vi "Redirect Versions in Deployment Project File.vi"() -> ()   [LabVIEW 2013, in "Assembly Redirection VIs.lvlib"]
uses:
  Assembly Redirection VIs.lvlib
panel:
  in  "New TestStand Registry Version":string="5.1"
  in  "New VeriStand Version":string="2013"
  in  "destination file path":path=path "C:/Users/achurch/Documents/Source/XML Assembly Redirection Project/Examples XML Files/VeristandStepsInstaller_mod.vdproj"
  out "error out":errorcluster
  in  "New TestStand Version":string="2013"
  in  "configuration file path":path=path "C:/Users/achurch/Documents/Source/XML Assembly Redirection Project/Examples XML Files/VeristandStepsInstaller.vdproj"
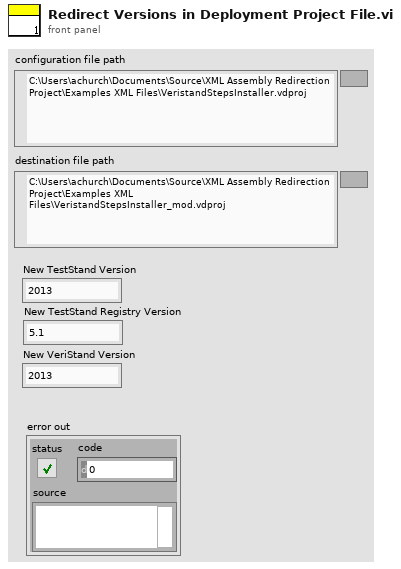
[diagram p1: front panel]
types:
  T1 = enum16{"open", "replace", "create", "open or create", "replace or create", "replace or create with confirmation"}
  T2 = enum32{"invalid app kind", "Development System", "Run Time System", "Student Edition", "Embedded LabVIEW", "Evaluation", "Custom"}
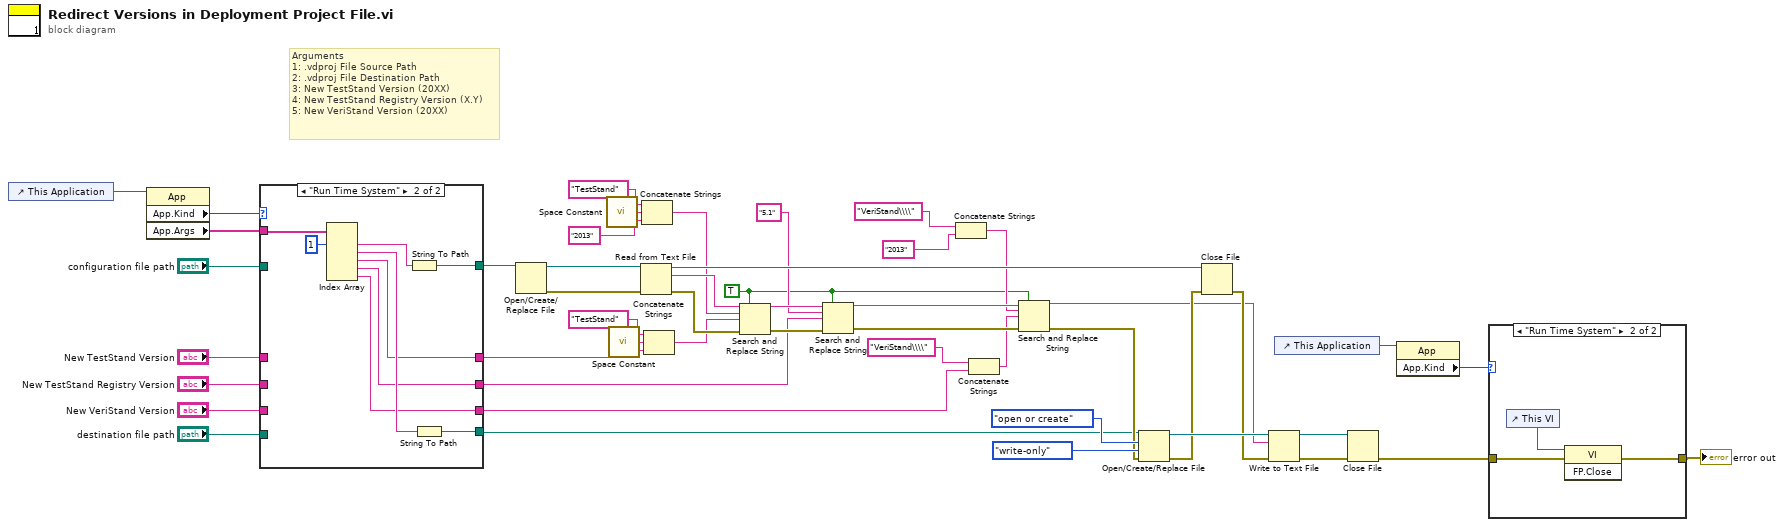
[diagram p0: block diagram]
diagram:
  w18 = TRUE ("replace all? (F)")
  # "Arguments\n1: .vdproj File Source Path\n2: .vdproj File Destination Path\n3: New TestStand Version (20XX)\n4: New TestStand Registry Version (X.Y)\n5: New VeriStand Version (20XX)"
  n1 = control-ref of="This Application"() -> (w17:refnum<vi>)
  n2 = property class="App"(reference=w17) -> ("App.Kind"=w16:T2, "App.Args"=w15:string[])  [unwired: 1 in, 2 out]
  n3 = case shown="\"Run Time System\"" w16 {
    tunnel: w15 -> [_ w63]
    tunnel: "configuration file path" -> [w50 _]
    tunnel: "New TestStand Version" -> [w54 _]
    tunnel: "New TestStand Registry Version" -> [w52 _]
    tunnel: "New VeriStand Version" -> [w51 _]
    tunnel: "destination file path" -> [w53 _]
    tunnel: [w50 w60] -> w9
    tunnel: [w53 w58] -> w5
    tunnel: [w54 w57] -> w8
    tunnel: [w52 w56] -> w7
    tunnel: [w51 w55] -> w6
    frame "Development System", Default {
    }
    frame "Run Time System" {
      n4 = Index Array(array=w63, index #1=1 ("index")) -> (element #1=w61:string, element #2=w59:string, element #3=w57:string, element #4=w56:string, element #5=w55:string)  [unwired: 4 in]
      n5 = String To Path(string=w61) -> (path=w60:path)
      n6 = String To Path(string=w59) -> (path=w58:path)
    }
  }
  n7 = Open/Create/Replace File(file path (use dialog)=w9) -> (refnum out=w48:refnum<file>, error out=w49:errorcluster)  [unwired: 5 in, 1 out]
  n8 = call <vilib>:"Space Constant.vi"() -> ("String"=w37:string)
  n9 = call <vilib>:"Space Constant.vi"() -> ("String"=w32:string)
  n10 = Read from Text File(file (use dialog)=w48, error in=w49) -> (refnum out=w45:refnum<file>, text=w46:string, error out=w47:errorcluster)  [unwired: 2 in, 1 out]
  n11 = Concatenate Strings("TestStand" ("search string"), w37, "2013" ("search string")) -> (w34:string)
  n12 = Concatenate Strings("TestStand" ("search string"), w32, w8) -> (w31:string)
  n13 = Search and Replace String(replace all?=w18, input string=w46, search string=w34, replace string=w31, error in=w47) -> (result string=w29:string, error out=w30:errorcluster)  [unwired: 3 in, 2 out]
  n14 = Search and Replace String(replace all?=w18, input string=w29, search string="5.1", replace string=w7, error in=w30) -> (result string=w26:string, error out=w27:errorcluster)  [unwired: 3 in, 2 out]
  n15 = Concatenate Strings("VeriStand\\\\" ("search string"), "2013" ("search string")) -> (w21:string)
  n16 = Concatenate Strings("VeriStand\\\\" ("search string"), w6) -> (w22:string)
  n17 = Search and Replace String(replace all?=w18, input string=w26, search string=w21, replace string=w22, error in=w27) -> (result string=w19:string, error out=w20:errorcluster)  [unwired: 3 in, 2 out]
  n18 = Open/Create/Replace File(file path (use dialog)=w5, error in=w20, operation (0:open)=T1."open or create", access (0:read/write)=enum16{"read/write", "read-only", "write-only"}."write-only") -> (refnum out=w42:refnum<file>, error out=w41:errorcluster)  [unwired: 2 in, 1 out]
  n19 = Close File(refnum=w45, error in=w41) -> (error out=w40:errorcluster)  [unwired: 1 out]
  n20 = Write to Text File(file (use dialog)=w42, text=w19, error in=w40) -> (refnum out=w38:refnum<file>, error out=w39:errorcluster)  [unwired: 1 in, 1 out]
  n21 = control-ref of="This Application"() -> (w4:refnum<vi>)
  n22 = Close File(refnum=w38, error in=w39) -> (error out=w2:errorcluster)  [unwired: 1 out]
  n23 = property class="App"(reference=w4) -> ("App.Kind"=w3:T2)  [unwired: 1 in, 2 out]
  n24 = case shown="\"Run Time System\"" w3 {
    tunnel: w2 -> [w64 w66]
    tunnel: [w64 w65] -> w1
    frame "Development System", Default {
    }
    frame "Run Time System" {
      n25 = control-ref of="This VI"() -> (w67:refnum<vi>)
      n26 = invoke class="VI" method="FP.Close"(reference=w67, error in=w66) -> (error out=w65:errorcluster)  [unwired: 1 in, 2 out]
    }
  }
  "error out" <- w1
